vi "Autonomous 1 container 1 tote.vi"() -> ()   [LabVIEW 2014]
uses:
  Control 3.ctl
  Robot Global Data.vi
panel:
  in  "Parameters":T1
  in  "IR Sensors":bool
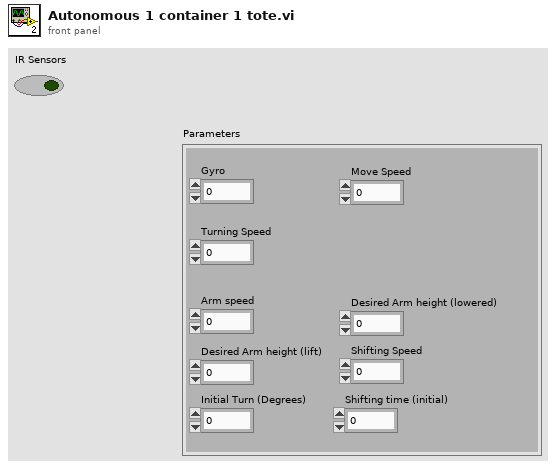
[diagram p1: front panel]
types:
  T1 = cluster{"Gyro":dbl, "Turning Speed":dbl, "Move Speed":dbl, "Arm speed":dbl, "Desired Arm height (lift)":dbl, "Initial Turn (Degrees)":dbl, "Desired Arm height (lowered)":dbl, "Shifting Speed":dbl, "Shifting time (initial)":dbl}
  T2 = typedef "Control 3.ctl" = enum16{"Start", "Grab container", "Lift arms", "Position robot", "Let go of container + Lower Arms", "Lift tote and container", "Shift Sideways", "Move Forward", "Shift to Auto Area", "Stop"}
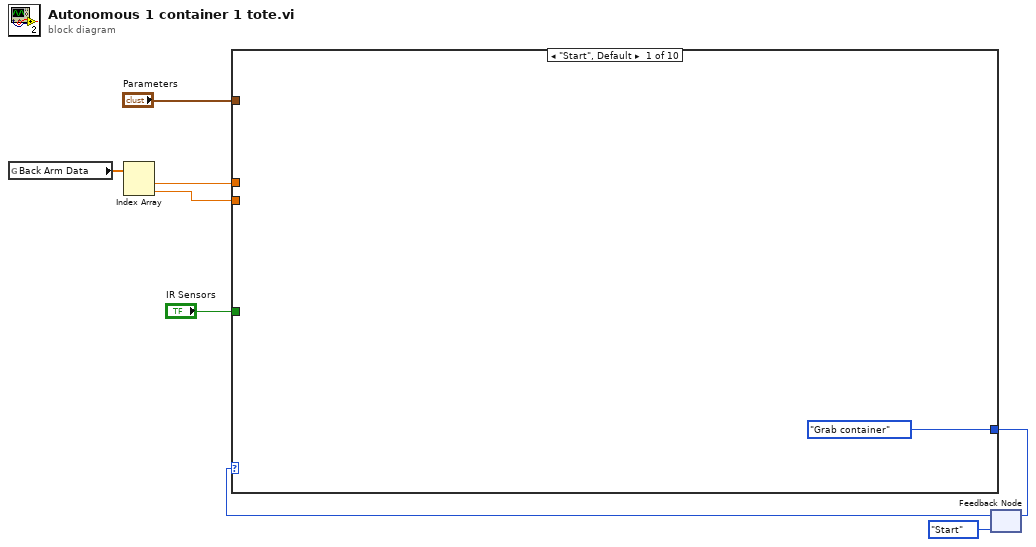
[diagram p0: block diagram]
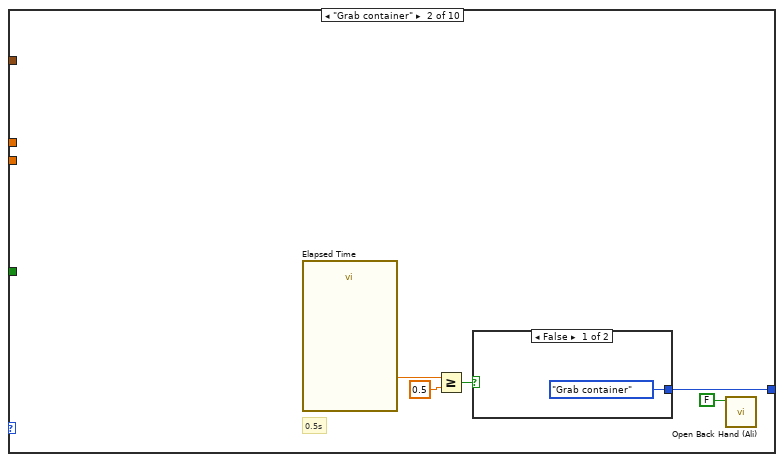
[diagram p2: hidden frame]
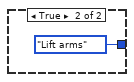
[diagram p3: hidden frame]
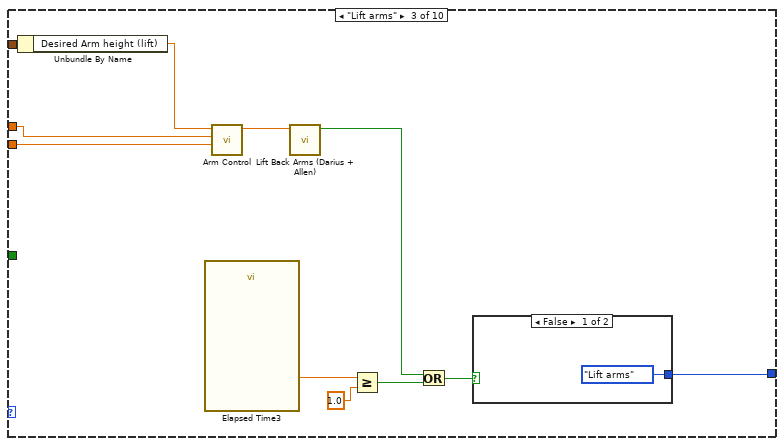
[diagram p4: hidden frame]
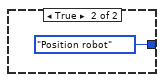
[diagram p5: hidden frame]
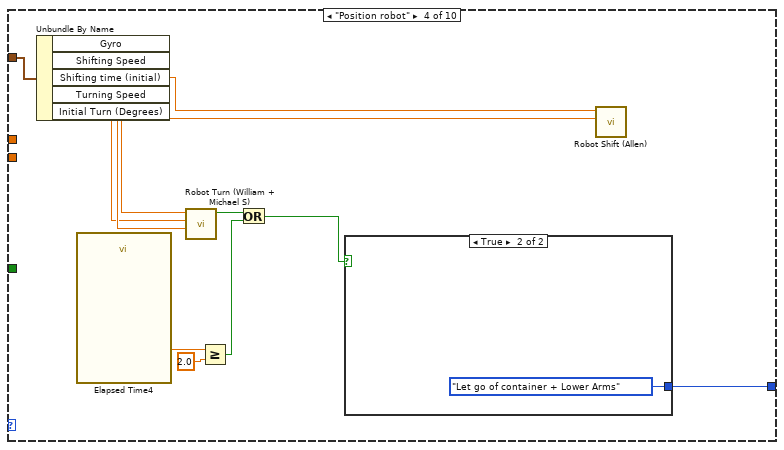
[diagram p6: hidden frame]
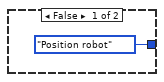
[diagram p7: hidden frame]
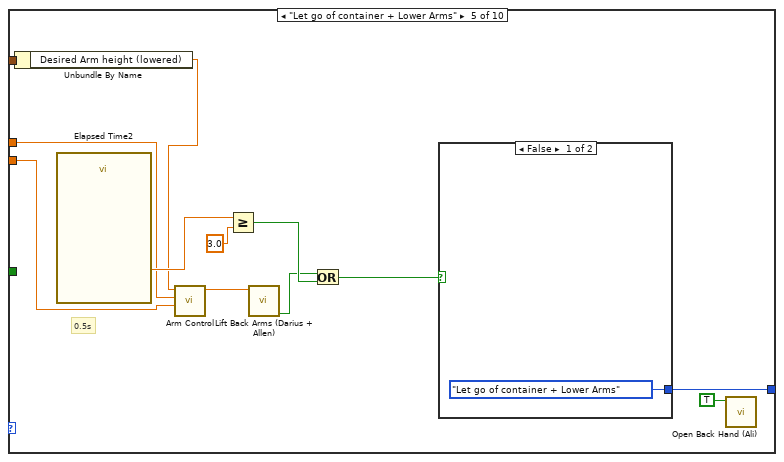
[diagram p8: hidden frame]
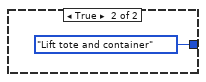
[diagram p9: hidden frame]
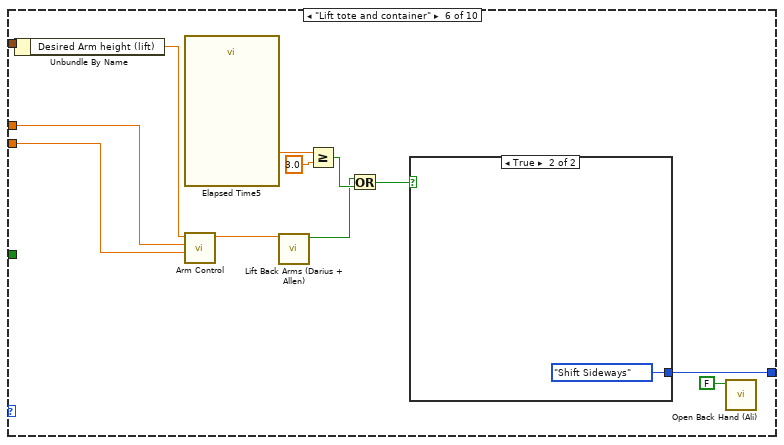
[diagram p10: hidden frame]
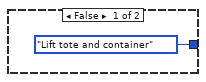
[diagram p11: hidden frame]
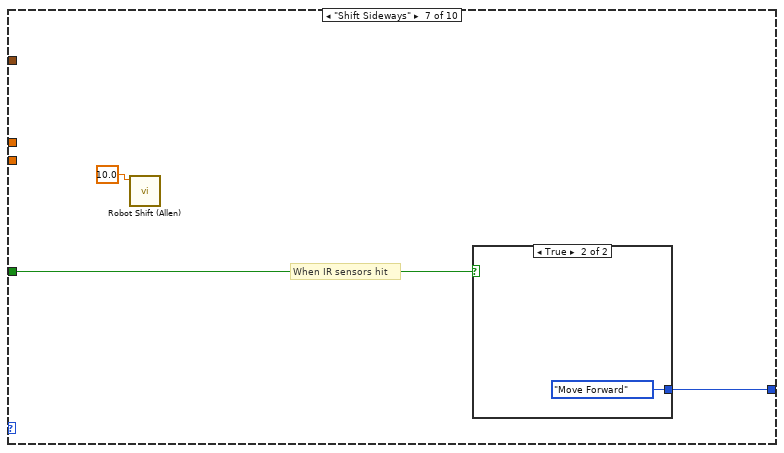
[diagram p12: hidden frame]
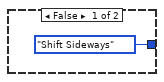
[diagram p13: hidden frame]
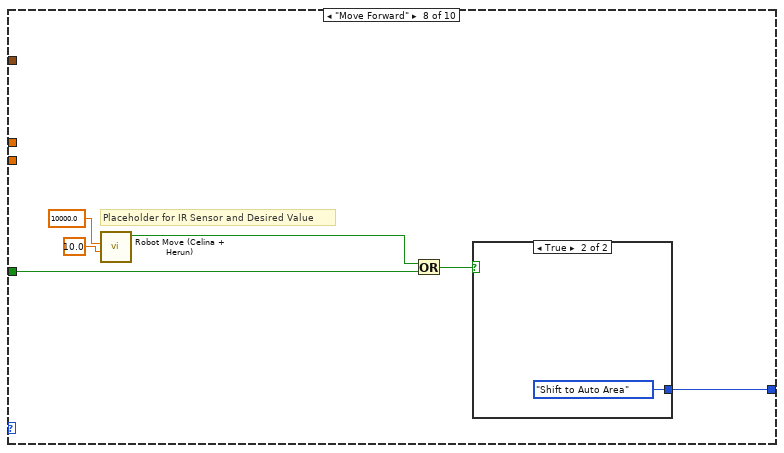
[diagram p14: hidden frame]
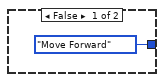
[diagram p15: hidden frame]
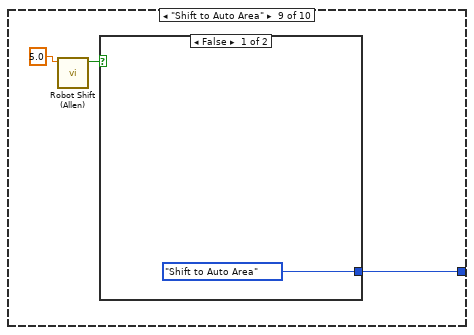
[diagram p16: hidden frame]
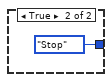
[diagram p17: hidden frame]
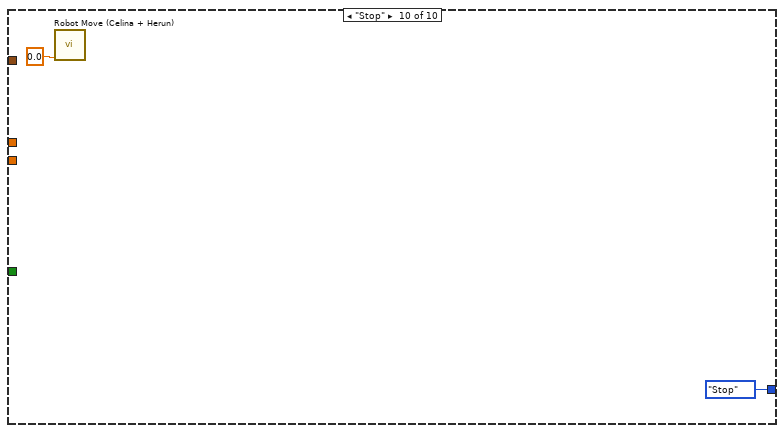
[diagram p18: hidden frame]
diagram:
  n1 = global read "Robot Global Data.vi" "Back Arm Data"() -> (w4:dbl[])
  n2 = Index Array(array=w4) -> (element #1=w3:dbl, element #2=w2:dbl)  [unwired: 2 in]
  n3 = feedback #1(Control_3."Start") -> (w8:T2)
  n4 = case shown="\"Start\", Default" w8 {
    tunnel: [Control_3."Grab container" w11 w23 w36 w52 w66 w74 w81 w87 Control_3."Stop"] -> w7
    tunnel: "IR Sensors" -> [_ _ _ _ _ _ w72 w79 _ _]
    tunnel: w3 -> [_ _ w18 _ w46 w59 _ _ _ _]
    tunnel: w2 -> [_ _ w17 _ w45 w58 _ _ _ _]
    tunnel: "Parameters" -> [_ _ w22 w35 w48 w63 _ _ _ _]
    frame "Start", Default {
    }
    frame "Grab container" {
      # "0.5s"
      n5 = call "Elapsed Time"() -> ("Elapsed Time (s)"=w14:dbl)  [unwired: 12 in, 7 out]
      n6 = Greater Or Equal?(x=w14, y=0.5) -> (x >= y?=w12:bool)
      n7 = case shown="False" w12 {
        tunnel: [Control_3."Grab container" Control_3."Lift arms"] -> w11
        frame False {
        }
        frame True {
        }
      }
      n8 = call "Open Back Hand (Ali).vi"("Open?"=FALSE) -> ()  [unwired: 11 in]
    }
    frame "Lift arms" {
      n9 = Unbundle By Name(w22) -> ("Desired Arm height (lift)"=w19:dbl)
      n10 = call "Elapsed Time3"() -> ("Elapsed Time (s)"=w27:dbl)  [unwired: 12 in, 7 out]
      n11 = call "Arm Control.vi"("Current Speed"=w17, "Current Height"=w18, "Desired Height"=w19) -> ("Motor Output"=w20:dbl)  [unwired: 7 in, 1 out]
      n12 = call "Lift Back Arms (Darius + Allen).vi"("Motor Output"=w20) -> ("BackArmTop"=w21:bool)  [unwired: 9 in, 1 out]
      n13 = Greater Or Equal?(x=w27, y=1.0) -> (x >= y?=w25:bool)
      n14 = Or(x=w21, y=w25) -> (x .or. y?=w24:bool)
      n15 = case shown="False" w24 {
        tunnel: [Control_3."Lift arms" Control_3."Position robot"] -> w23
        frame False {
        }
        frame True {
        }
      }
    }
    frame "Position robot" {
      n16 = Unbundle By Name(w35) -> ("Gyro"=w34:dbl, "Shifting Speed"=w33:dbl, "Shifting time (initial)"=w32:dbl, "Turning Speed"=w31:dbl, "Initial Turn (Degrees)"=w30:dbl)
      n17 = call "Elapsed Time4"() -> ("Elapsed Time (s)"=w41:dbl)  [unwired: 12 in, 7 out]
      n18 = call "Robot Turn (William + Michael S).vi"("X axis value"=w31, "Desired Degree"=w30, "Gyro Degrees"=w34) -> ("Stop"=w39:bool)  [unwired: 8 in]
      n19 = Greater Or Equal?(x=w41, y=2.0) -> (x >= y?=w38:bool)
      n20 = Or(x=w39, y=w38) -> (x .or. y?=w37:bool)
      n21 = case shown="True" w37 {
        tunnel: [Control_3."Position robot" Control_3."Let go of container + Lower Arms"] -> w36
        frame False {
        }
        frame True {
        }
      }
      n22 = call "Robot Shift (Allen).vi"("speed"=w33, "Move time"=w32) -> ()  [unwired: 9 in, 1 out]
    }
    frame "Let go of container + Lower Arms" {
      # "0.5s"
      n23 = Unbundle By Name(w48) -> ("Desired Arm height (lowered)"=w44:dbl)
      n24 = call "Elapsed Time2"() -> ("Elapsed Time (s)"=w53:dbl)  [unwired: 12 in, 7 out]
      n25 = call "Arm Control.vi"("Current Speed"=w45, "Current Height"=w46, "Desired Height"=w44) -> ("Motor Output"=w47:dbl)  [unwired: 7 in, 1 out]
      n26 = Greater Or Equal?(x=w53, y=3.0) -> (x >= y?=w55:bool)
      n27 = call "Lift Back Arms (Darius + Allen).vi"("Motor Output"=w47) -> ("BackArmBottom"=w50:bool)  [unwired: 9 in, 1 out]
      n28 = Or(x=w50, y=w55) -> (x .or. y?=w49:bool)
      n29 = case shown="False" w49 {
        tunnel: [Control_3."Let go of container + Lower Arms" Control_3."Lift tote and container"] -> w52
        frame False {
        }
        frame True {
        }
      }
      n30 = call "Open Back Hand (Ali).vi"("Open?"=TRUE) -> ()  [unwired: 11 in]
    }
    frame "Lift tote and container" {
      n31 = Unbundle By Name(w63) -> ("Desired Arm height (lift)"=w60:dbl)
      n32 = call "Elapsed Time5"() -> ("Elapsed Time (s)"=w68:dbl)  [unwired: 12 in, 7 out]
      n33 = call "Arm Control.vi"("Current Speed"=w58, "Current Height"=w59, "Desired Height"=w60) -> ("Motor Output"=w61:dbl)  [unwired: 7 in, 1 out]
      n34 = call "Lift Back Arms (Darius + Allen).vi"("Motor Output"=w61) -> ("BackArmTop"=w62:bool)  [unwired: 9 in, 1 out]
      n35 = Greater Or Equal?(x=w68, y=3.0) -> (x >= y?=w65:bool)
      n36 = Or(x=w62, y=w65) -> (x .or. y?=w64:bool)
      n37 = case shown="True" w64 {
        tunnel: [Control_3."Lift tote and container" Control_3."Shift Sideways"] -> w66
        frame False {
        }
        frame True {
        }
      }
      n38 = call "Open Back Hand (Ali).vi"("Open?"=FALSE) -> ()  [unwired: 11 in]
    }
    frame "Shift Sideways" {
      # "When IR sensors hit"
      n39 = call "Robot Shift (Allen).vi"("Move time"=10.0) -> ()  [unwired: 10 in, 1 out]
      n40 = case shown="True" w72 {
        tunnel: [Control_3."Shift Sideways" Control_3."Move Forward"] -> w74
        frame False {
        }
        frame True {
        }
      }
    }
    frame "Move Forward" {
      # "Placeholder for IR Sensor and Desired Value"
      n41 = call "Robot Move (Celina + Herun).vi"("Desired Time"=10.0, "Desired Distance (ft)"=10000.0) -> ("Stop State"=w80:bool)  [unwired: 9 in]
      n42 = Or(x=w80, y=w79) -> (x .or. y?=w78:bool)
      n43 = case shown="True" w78 {
        tunnel: [Control_3."Move Forward" Control_3."Shift to Auto Area"] -> w81
        frame False {
        }
        frame True {
        }
      }
    }
    frame "Shift to Auto Area" {
      n44 = call "Robot Shift (Allen).vi"("Move time"=5.0) -> ("Done"=w86:bool)  [unwired: 10 in]
      n45 = case shown="False" w86 {
        tunnel: [Control_3."Shift to Auto Area" Control_3."Stop"] -> w87
        frame False {
        }
        frame True {
        }
      }
    }
    frame "Stop" {
      n46 = call "Robot Move (Celina + Herun).vi"("Y axis value"=0.0) -> ()  [unwired: 10 in, 1 out]
    }
  }
  n47 = feedback-in #1(w7) -> ()
